vi "FeedbackDecode.vi"() -> ()   [LabVIEW 2020] (continued)
            n2364 = call "FeedbackDecode_MLComCtrl.vi"("DecodeClustIn"=w2568, "Mode"=T19."SendEvent") -> ()  [unwired: 6 in, 4 out]
          }
          event Value Change {
            n2365 = event-data() -> ()  [unwired: 1 in, 6 out]
            n2366 = local read "EncodeClust"() -> (w2595:T9)
            n2367 = call "FeedbackDecode_BuildStimCmd.vi"("EncodeClustIn"=w2595) -> ("EncodeClustOut"=w2594:T9, "StimCmd"=w2579:string)  [unwired: 1 in]
            n2368 = local read "LoopCnt"() -> (w2589:u64)
            n2369 = local write "EncodeClust"(w2594) -> ()
            n2370 = local read "NIPTime"() -> (w2585:dbl)
            n2371 = Format Into String(w2589) -> (resulting string=w2580:string)  [unwired: 3 in, 1 out]
            n2372 = call-poly "FeedbackDecode_VariablesToString.vi"("Format"="%0.0f", "ValueIn"=w2585, "FieldName"="NIPTime" ("Key Word")) -> ("StringOut"=w2582:string)  [unwired: 4 in]
            n2373 = local read "EventParamsFID"() -> (w2592:refnum<file>)
            n2374 = Concatenate Strings("ChangeJitter:SS.EventID=" ("string"), w2580) -> (w2588:string)
            n2375 = local write "StimCmd"(w2579) -> ()
            n2376 = Concatenate Strings(w2588, ";", w2579, w2582) -> (w2587:string)
            n2377 = local read "DecodeClust"() -> (w2593:T5)
            n2378 = call "FeedbackDecode_WriteTextEOL.vi"("text"=w2587, "refnum in"=w2592) -> ()  [unwired: 8 in, 2 out]
            n2379 = Bundle By Name(cluster=w2593, "EventStr"=w2587) -> (w2586:T5)
            n2380 = call "FeedbackDecode_MLComCtrl.vi"("DecodeClustIn"=w2586, "Mode"=T19."SendEvent") -> ()  [unwired: 6 in, 4 out]
          }
          event Value Change {
            n2381 = event-data() -> ()  [unwired: 1 in, 6 out]
            n2382 = local read "EncodeClust"() -> (w2613:T9)
            n2383 = call "FeedbackDecode_BuildStimCmd.vi"("EncodeClustIn"=w2613) -> ("EncodeClustOut"=w2612:T9, "StimCmd"=w2597:string)  [unwired: 1 in]
            n2384 = local read "LoopCnt"() -> (w2607:u64)
            n2385 = local write "EncodeClust"(w2612) -> ()
            n2386 = local read "NIPTime"() -> (w2603:dbl)
            n2387 = Format Into String(w2607) -> (resulting string=w2598:string)  [unwired: 3 in, 1 out]
            n2388 = call-poly "FeedbackDecode_VariablesToString.vi"("Format"="%0.0f", "ValueIn"=w2603, "FieldName"="NIPTime" ("Key Word")) -> ("StringOut"=w2600:string)  [unwired: 4 in]
            n2389 = Concatenate Strings("ChangeBFreq:SS.EventID=" ("string"), w2598) -> (w2606:string)
            n2390 = local read "EventParamsFID"() -> (w2610:refnum<file>)
            n2391 = local write "StimCmd"(w2597) -> ()
            n2392 = Concatenate Strings(w2606, ";", w2597, w2600) -> (w2605:string)
            n2393 = local read "DecodeClust"() -> (w2611:T5)
            n2394 = call "FeedbackDecode_WriteTextEOL.vi"("text"=w2605, "refnum in"=w2610) -> ()  [unwired: 8 in, 2 out]
            n2395 = Bundle By Name(cluster=w2611, "EventStr"=w2605) -> (w2604:T5)
            n2396 = call "FeedbackDecode_MLComCtrl.vi"("DecodeClustIn"=w2604, "Mode"=T19."SendEvent") -> ()  [unwired: 6 in, 4 out]
          }
          event Value Change {
            n2397 = event-data() -> ()  [unwired: 1 in, 6 out]
            n2398 = local read "EncodeClust"() -> (w2631:T9)
            n2399 = call "FeedbackDecode_BuildStimCmd.vi"("EncodeClustIn"=w2631) -> ("EncodeClustOut"=w2630:T9, "StimCmd"=w2615:string)  [unwired: 1 in]
            n2400 = local read "LoopCnt"() -> (w2625:u64)
            n2401 = local write "EncodeClust"(w2630) -> ()
            n2402 = local read "NIPTime"() -> (w2621:dbl)
            n2403 = Format Into String(w2625) -> (resulting string=w2616:string)  [unwired: 3 in, 1 out]
            n2404 = call-poly "FeedbackDecode_VariablesToString.vi"("Format"="%0.0f", "ValueIn"=w2621, "FieldName"="NIPTime" ("Key Word")) -> ("StringOut"=w2618:string)  [unwired: 4 in]
            n2405 = local read "EventParamsFID"() -> (w2628:refnum<file>)
            n2406 = Concatenate Strings("ChangeBAmp:SS.EventID=" ("string"), w2616) -> (w2624:string)
            n2407 = local write "StimCmd"(w2615) -> ()
            n2408 = local read "DecodeClust"() -> (w2629:T5)
            n2409 = Concatenate Strings(w2624, ";", w2615, w2618) -> (w2623:string)
            n2410 = call "FeedbackDecode_WriteTextEOL.vi"("text"=w2623, "refnum in"=w2628) -> ()  [unwired: 8 in, 2 out]
            n2411 = Bundle By Name(cluster=w2629, "EventStr"=w2623) -> (w2622:T5)
            n2412 = call "FeedbackDecode_MLComCtrl.vi"("DecodeClustIn"=w2622, "Mode"=T19."SendEvent") -> ()  [unwired: 6 in, 4 out]
          }
          event "TASKA Shared Control": Value Change {
            n2413 = event-data() -> ("NewVal"=w2635:bool)  [unwired: 1 in, 5 out]
            n2414 = case shown="True" w2635 {
              tunnel: [0.0 1.0] -> w2634
              frame False {
              }
              frame True {
              }
            }
            n2415 = local read "LoopCnt"() -> (w2644:u64)
            n2416 = call-poly "FeedbackDecode_VariablesToString.vi"("Format"="%d", "ValueIn"=w2634, "FieldName"="TASKASensors.SharedControl.Ready") -> ("StringOut"=w2651:string)  [unwired: 4 in]
            n2417 = local read "NIPTime"() -> (w2640:dbl)
            n2418 = Format Into String(w2644) -> (resulting string=w2636:string)  [unwired: 3 in, 1 out]
            n2419 = local read "EventParamsFID"() -> (w2648:refnum<file>)
            n2420 = local read "DecodeClust"() -> (w2649:T5)
            n2421 = Concatenate Strings("SharedControl:SS.EventID=" ("string"), w2636) -> (w2643:string)
            n2422 = call-poly "FeedbackDecode_VariablesToString.vi"("Format"="%0.0f", "ValueIn"=w2640, "FieldName"="NIPTime" ("Key Word")) -> ("StringOut"=w2637:string)  [unwired: 4 in]
            n2423 = Concatenate Strings(w2643, ";", w2651, w2637) -> (w2642:string)
            n2424 = call "FeedbackDecode_WriteTextEOL.vi"("text"=w2642, "refnum in"=w2648) -> ()  [unwired: 8 in, 2 out]
            n2425 = Bundle By Name(cluster=w2649, "EventStr"=w2642) -> (w2641:T5)
            n2426 = call "FeedbackDecode_MLComCtrl.vi"("DecodeClustIn"=w2641, "Mode"=T19."SendEvent") -> ()  [unwired: 6 in, 4 out]
          }
          event "TASKA Timer": Value Change {
            n2427 = event-data() -> ("NewVal"=w2655:bool)  [unwired: 1 in, 5 out]
            n2428 = case shown="True" w2655 {
              frame True {
                n2429 = local read "LoopCnt"() -> (w2660:u64)
                n2430 = local read "NIPTime"() -> (w2663:dbl)
                n2431 = Format Into String(w2660) -> (resulting string=w2667:string)  [unwired: 3 in, 1 out]
                n2432 = local read "EventParamsFID"() -> (w2657:refnum<file>)
                n2433 = Concatenate Strings("SharedControlStartTime:SS.EventID=" ("string"), w2667) -> (w2661:string)
                n2434 = call-poly "FeedbackDecode_VariablesToString.vi"("Format"="%0.0f", "ValueIn"=w2663, "FieldName"="NIPTime" ("Key Word")) -> ("StringOut"=w2666:string)  [unwired: 4 in]
                n2435 = Concatenate Strings(w2661, ";", w2666) -> (w2662:string)
                n2436 = call "FeedbackDecode_WriteTextEOL.vi"("text"=w2662, "refnum in"=w2657) -> ()  [unwired: 8 in, 2 out]
              }
              frame False {
                n2437 = property on="TASKA Timer" class="Bool (strict)"("DisabledEnum"=T17."Disabled and Grayed Out" ("Disabled")) -> ()  [unwired: 2 in, 2 out]
                n2438 = local read "LoopCnt"() -> (w2672:u64)
                n2439 = local read "NIPTime"() -> (w2675:dbl)
                n2440 = Format Into String(w2672) -> (resulting string=w2679:string)  [unwired: 3 in, 1 out]
                n2441 = local read "EventParamsFID"() -> (w2669:refnum<file>)
                n2442 = Concatenate Strings("SharedControlStopTime:SS.EventID=" ("string"), w2679) -> (w2673:string)
                n2443 = call-poly "FeedbackDecode_VariablesToString.vi"("Format"="%0.0f", "ValueIn"=w2675, "FieldName"="NIPTime" ("Key Word")) -> ("StringOut"=w2678:string)  [unwired: 4 in]
                n2444 = Concatenate Strings(w2673, ";", w2678) -> (w2674:string)
                n2445 = call "FeedbackDecode_WriteTextEOL.vi"("text"=w2674, "refnum in"=w2669) -> ()  [unwired: 8 in, 2 out]
              }
            }
          }
          event "TASKA Reset Break": Value Change {
            n2446 = event-data() -> ()  [unwired: 1 in, 6 out]
            n2447 = call-poly "FeedbackDecode_VariablesToString.vi"("Format"="%0.0f", "ValueIn"=0.0, "FieldName"="SharedControlTrialSuccess" ("Key Word")) -> ("StringOut"=w2681:string)  [unwired: 4 in]
            n2448 = property on="TASKA Timer" class="Bool (strict)"("DisabledEnum"=T17."Enabled" ("Disabled")) -> ()  [unwired: 2 in, 2 out]
            n2449 = local read "LoopCnt"() -> (w2688:u64)
            n2450 = local read "NIPTime"() -> (w2691:dbl)
            n2451 = Format Into String(w2688) -> (resulting string=w2695:string)  [unwired: 3 in, 1 out]
            n2452 = local read "EventParamsFID"() -> (w2685:refnum<file>)
            n2453 = Concatenate Strings("SharedControlTrialResult:SS.EventID=" ("string"), w2695) -> (w2689:string)
            n2454 = call-poly "FeedbackDecode_VariablesToString.vi"("Format"="%0.0f", "ValueIn"=w2691, "FieldName"="NIPTime" ("Key Word")) -> ("StringOut"=w2694:string)  [unwired: 4 in]
            n2455 = Concatenate Strings(w2689, ";", w2681, w2694) -> (w2690:string)
            n2456 = call "FeedbackDecode_WriteTextEOL.vi"("text"=w2690, "refnum in"=w2685) -> ()  [unwired: 8 in, 2 out]
          }
          event "TASKA Reset Success": Value Change {
            n2457 = event-data() -> ()  [unwired: 1 in, 6 out]
            n2458 = call-poly "FeedbackDecode_VariablesToString.vi"("Format"="%0.0f", "ValueIn"=1.0, "FieldName"="SharedControlTrialSuccess" ("Key Word")) -> ("StringOut"=w2698:string)  [unwired: 4 in]
            n2459 = property on="TASKA Timer" class="Bool (strict)"("DisabledEnum"=T17."Enabled" ("Disabled")) -> ()  [unwired: 2 in, 2 out]
            n2460 = local read "LoopCnt"() -> (w2705:u64)
            n2461 = local read "NIPTime"() -> (w2708:dbl)
            n2462 = Format Into String(w2705) -> (resulting string=w2712:string)  [unwired: 3 in, 1 out]
            n2463 = local read "EventParamsFID"() -> (w2702:refnum<file>)
            n2464 = Concatenate Strings("SharedControlTrialResult:SS.EventID=" ("string"), w2712) -> (w2706:string)
            n2465 = call-poly "FeedbackDecode_VariablesToString.vi"("Format"="%0.0f", "ValueIn"=w2708, "FieldName"="NIPTime" ("Key Word")) -> ("StringOut"=w2711:string)  [unwired: 4 in]
            n2466 = Concatenate Strings(w2706, ";", w2698, w2711) -> (w2707:string)
            n2467 = call "FeedbackDecode_WriteTextEOL.vi"("text"=w2707, "refnum in"=w2702) -> ()  [unwired: 8 in, 2 out]
          }
          event "TASKASharedControlBeta": Value Change {
            n2468 = event-data() -> ("NewVal"=w2714:dbl)  [unwired: 1 in, 5 out]
            n2469 = local read "LoopCnt"() -> (w2724:u64)
            n2470 = call-poly "FeedbackDecode_VariablesToString.vi"("Format"="%0.5f", "ValueIn"=w2714, "FieldName"="TASKASensors.SharedControl.Beta") -> ("StringOut"=w2731:string)  [unwired: 4 in]
            n2471 = local read "NIPTime"() -> (w2720:dbl)
            n2472 = Format Into String(w2724) -> (resulting string=w2716:string)  [unwired: 3 in, 1 out]
            n2473 = local read "EventParamsFID"() -> (w2728:refnum<file>)
            n2474 = local read "DecodeClust"() -> (w2729:T5)
            n2475 = Concatenate Strings("SharedControl:SS.EventID=" ("string"), w2716) -> (w2723:string)
            n2476 = call-poly "FeedbackDecode_VariablesToString.vi"("Format"="%0.0f", "ValueIn"=w2720, "FieldName"="NIPTime" ("Key Word")) -> ("StringOut"=w2717:string)  [unwired: 4 in]
            n2477 = Concatenate Strings(w2723, ";", w2731, w2717) -> (w2722:string)
            n2478 = call "FeedbackDecode_WriteTextEOL.vi"("text"=w2722, "refnum in"=w2728) -> ()  [unwired: 8 in, 2 out]
            n2479 = Bundle By Name(cluster=w2729, "EventStr"=w2722) -> (w2721:T5)
            n2480 = call "FeedbackDecode_MLComCtrl.vi"("DecodeClustIn"=w2721, "Mode"=T19."SendEvent") -> ()  [unwired: 6 in, 4 out]
          }
          event "TASKASharedControlIncrememnt": Value Change {
            n2481 = event-data() -> ("NewVal"=w2733:dbl)  [unwired: 1 in, 5 out]
            n2482 = local read "LoopCnt"() -> (w2743:u64)
            n2483 = call-poly "FeedbackDecode_VariablesToString.vi"("Format"="%0.5f", "ValueIn"=w2733, "FieldName"="TASKASensors.SharedControl.Increment") -> ("StringOut"=w2750:string)  [unwired: 4 in]
            n2484 = local read "NIPTime"() -> (w2739:dbl)
            n2485 = Format Into String(w2743) -> (resulting string=w2735:string)  [unwired: 3 in, 1 out]
            n2486 = local read "EventParamsFID"() -> (w2747:refnum<file>)
            n2487 = local read "DecodeClust"() -> (w2748:T5)
            n2488 = Concatenate Strings("SharedControl:SS.EventID=" ("string"), w2735) -> (w2742:string)
            n2489 = call-poly "FeedbackDecode_VariablesToString.vi"("Format"="%0.0f", "ValueIn"=w2739, "FieldName"="NIPTime" ("Key Word")) -> ("StringOut"=w2736:string)  [unwired: 4 in]
            n2490 = Concatenate Strings(w2742, ";", w2750, w2736) -> (w2741:string)
            n2491 = call "FeedbackDecode_WriteTextEOL.vi"("text"=w2741, "refnum in"=w2747) -> ()  [unwired: 8 in, 2 out]
            n2492 = Bundle By Name(cluster=w2748, "EventStr"=w2741) -> (w2740:T5)
            n2493 = call "FeedbackDecode_MLComCtrl.vi"("DecodeClustIn"=w2740, "Mode"=T19."SendEvent") -> ()  [unwired: 6 in, 4 out]
          }
          event "IndexSet", "MiddleSet", "RingSet", "PinkySet", "ThumbSet", "ThumbIntSet": Value Change {
            n2494 = event-data() -> ()  [unwired: 1 in, 6 out]
            n2495 = local read "ThumbIntSet"() -> (w2752:dbl)
            n2496 = local read "ThumbSet"() -> (w2753:dbl)
            n2497 = local read "MiddleSet"() -> (w2758:dbl)
            n2498 = local read "RingSet"() -> (w2757:dbl)
            n2499 = local read "PinkySet"() -> (w2754:dbl)
            n2500 = local read "IndexSet"() -> (w2759:dbl)
            n2501 = Build Array(w2759, w2758, w2757, w2754, w2753, w2752) -> (w2756:dbl[])
            n2502 = local read "LoopCnt"() -> (w2768:u64)
            n2503 = call-poly "FeedbackDecode_VariablesToString.vi"("Format"="%0.5f", "ValueIn"=w2756, "FieldName"="TASKA.RestPositions") -> ("StringOut"=w2775:string)  [unwired: 4 in]
            n2504 = local read "NIPTime"() -> (w2764:dbl)
            n2505 = Format Into String(w2768) -> (resulting string=w2761:string)  [unwired: 3 in, 1 out]
            n2506 = local read "EventParamsFID"() -> (w2772:refnum<file>)
            n2507 = local read "DecodeClust"() -> (w2773:T5)
            n2508 = Concatenate Strings("SharedControl:SS.EventID=" ("string"), w2761) -> (w2767:string)
            n2509 = call-poly "FeedbackDecode_VariablesToString.vi"("Format"="%0.0f", "ValueIn"=w2764, "FieldName"="NIPTime" ("Key Word")) -> ("StringOut"=w2755:string)  [unwired: 4 in]
            n2510 = Concatenate Strings(w2767, ";", w2775, w2755) -> (w2766:string)
            n2511 = call "FeedbackDecode_WriteTextEOL.vi"("text"=w2766, "refnum in"=w2772) -> ()  [unwired: 8 in, 2 out]
            n2512 = Bundle By Name(cluster=w2773, "EventStr"=w2766) -> (w2765:T5)
            n2513 = call "FeedbackDecode_MLComCtrl.vi"("DecodeClustIn"=w2765, "Mode"=T19."SendEvent") -> ()  [unwired: 6 in, 4 out]
          }
          event "ThumbShare", "IndexShare", "MiddleShare", "RingShare": Value Change {
            n2514 = event-data() -> ()  [unwired: 1 in, 6 out]
            n2515 = local read "ThumbShare"() -> (w2780:bool)
            n2516 = local read "MiddleShare"() -> (w2784:bool)
            n2517 = local read "RingShare"() -> (w2783:bool)
            n2518 = local read "IndexShare"() -> (w2785:bool)
            n2519 = Build Array(w2785, w2784, w2783, FALSE ("element"), w2780, FALSE ("element")) -> (w2778:bool[])
            n2520 = for {
              tunnel: w2778 -> [w2804] mode=indexing
              tunnel: [w2803] -> w2777 mode=indexing
              n2521 = case shown="False" w2804 {
                tunnel: [0.0 ("ValueIn") 1.0 ("ValueIn")] -> w2803
                frame False {
                }
                frame True {
                }
              }
            }
            n2522 = local read "LoopCnt"() -> (w2794:u64)
            n2523 = local read "NIPTime"() -> (w2790:dbl)
            n2524 = call-poly "FeedbackDecode_VariablesToString.vi"("Format"="%1.0f", "ValueIn"=w2777, "FieldName"="TASKASensors.SharedEnabled") -> ("StringOut"=w2801:string)  [unwired: 4 in]
            n2525 = Format Into String(w2794) -> (resulting string=w2787:string)  [unwired: 3 in, 1 out]
            n2526 = local read "EventParamsFID"() -> (w2798:refnum<file>)
            n2527 = local read "DecodeClust"() -> (w2799:T5)
            n2528 = Concatenate Strings("SharedControl:SS.EventID=" ("string"), w2787) -> (w2793:string)
            n2529 = call-poly "FeedbackDecode_VariablesToString.vi"("Format"="%0.0f", "ValueIn"=w2790, "FieldName"="NIPTime" ("Key Word")) -> ("StringOut"=w2782:string)  [unwired: 4 in]
            n2530 = Concatenate Strings(w2793, ";", w2801, w2782) -> (w2792:string)
            n2531 = call "FeedbackDecode_WriteTextEOL.vi"("text"=w2792, "refnum in"=w2798) -> ()  [unwired: 8 in, 2 out]
            n2532 = Bundle By Name(cluster=w2799, "EventStr"=w2792) -> (w2791:T5)
            n2533 = call "FeedbackDecode_MLComCtrl.vi"("DecodeClustIn"=w2791, "Mode"=T19."SendEvent") -> ()  [unwired: 6 in, 4 out]
          }
          event "Computer Goal": Value Change {
            n2534 = event-data() -> ("NewVal"=w2807:string)  [unwired: 1 in, 5 out]
            n2535 = local read "LoopCnt"() -> (w2817:u64)
            n2536 = call-poly "FeedbackDecode_VariablesToString.vi"("Format"="%0.5f", "ValueIn"=w2807, "FieldName"="TASKASensors.SharedControl.ComputerGoal") -> ("StringOut"=w2824:string)  [unwired: 4 in]
            n2537 = local read "NIPTime"() -> (w2813:dbl)
            n2538 = Format Into String(w2817) -> (resulting string=w2809:string)  [unwired: 3 in, 1 out]
            n2539 = local read "EventParamsFID"() -> (w2821:refnum<file>)
            n2540 = local read "DecodeClust"() -> (w2822:T5)
            n2541 = Concatenate Strings("SharedControl:SS.EventID=" ("string"), w2809) -> (w2816:string)
            n2542 = call-poly "FeedbackDecode_VariablesToString.vi"("Format"="%0.0f", "ValueIn"=w2813, "FieldName"="NIPTime" ("Key Word")) -> ("StringOut"=w2810:string)  [unwired: 4 in]
            n2543 = Concatenate Strings(w2816, ";", w2824, w2810) -> (w2815:string)
            n2544 = call "FeedbackDecode_WriteTextEOL.vi"("text"=w2815, "refnum in"=w2821) -> ()  [unwired: 8 in, 2 out]
            n2545 = Bundle By Name(cluster=w2822, "EventStr"=w2815) -> (w2814:T5)
            n2546 = call "FeedbackDecode_MLComCtrl.vi"("DecodeClustIn"=w2814, "Mode"=T19."SendEvent") -> ()  [unwired: 6 in, 4 out]
          }
          event "Beta Mode": Value Change {
            n2547 = event-data() -> ("NewVal"=w2826:string)  [unwired: 1 in, 5 out]
            n2548 = local read "LoopCnt"() -> (w2836:u64)
            n2549 = call-poly "FeedbackDecode_VariablesToString.vi"("Format"="%0.5f", "ValueIn"=w2826, "FieldName"="TASKASensors.SharedControl.BetaMode") -> ("StringOut"=w2843:string)  [unwired: 4 in]
            n2550 = local read "NIPTime"() -> (w2832:dbl)
            n2551 = Format Into String(w2836) -> (resulting string=w2828:string)  [unwired: 3 in, 1 out]
            n2552 = local read "EventParamsFID"() -> (w2840:refnum<file>)
            n2553 = local read "DecodeClust"() -> (w2841:T5)
            n2554 = Concatenate Strings("SharedControl:SS.EventID=" ("string"), w2828) -> (w2835:string)
            n2555 = call-poly "FeedbackDecode_VariablesToString.vi"("Format"="%0.0f", "ValueIn"=w2832, "FieldName"="NIPTime" ("Key Word")) -> ("StringOut"=w2829:string)  [unwired: 4 in]
            n2556 = Concatenate Strings(w2835, ";", w2843, w2829) -> (w2834:string)
            n2557 = call "FeedbackDecode_WriteTextEOL.vi"("text"=w2834, "refnum in"=w2840) -> ()  [unwired: 8 in, 2 out]
            n2558 = Bundle By Name(cluster=w2841, "EventStr"=w2834) -> (w2833:T5)
            n2559 = call "FeedbackDecode_MLComCtrl.vi"("DecodeClustIn"=w2833, "Mode"=T19."SendEvent") -> ()  [unwired: 6 in, 4 out]
          }
          event Mouse Wheel; Mouse Down; Mouse Move {
            n2560 = event-data() -> ("CtlRef"=w2845:refnum<vi>)  [unwired: 1 in, 4 out]
            n2561 = property class="Arr (strict)"(reference=w2845) -> ("Index Values"=w2846:u32[])  [unwired: 1 in, 2 out]
            n2562 = Index Array(array=w2846) -> (element=w2847:u32)  [unwired: 1 in]
            n2563 = Build Array(w2847) -> (w2848:u32[])
            n2564 = property on="Sel" class="Arr (strict)"("Index Values"=w2848) -> ()  [unwired: 2 in, 2 out]
          }
          event "RespStr": Value Change {
            n2565 = event-data() -> ("NewVal"=w2850:string)  [unwired: 1 in, 5 out]
            n2566 = Empty String/Path?(string/path=w2850) -> (empty?=w2851:bool)
            n2567 = case shown="False" w2851 {
              tunnel: w2850 -> [w2855 _]
              frame False {
                n2568 = xnode "Match Regular Expression"("input string"=w2855, "regular expression"="Sensor='") -> ("after match"=w2858:string)  [unwired: 4 in, 4 out]
                n2569 = local read "EncodeClust"() -> (w2860:T9)
                n2570 = xnode "Match Regular Expression"("input string"=w2858, "regular expression"="';") -> ("before match"=w2854:string)  [unwired: 4 in, 4 out]
                n2571 = call "FeedbackDecode_UpdateRegion.vi"("EncodeClustIn"=w2860, "RegionStr"=w2854) -> ("EncodeClustOut"=w2859:T9)  [unwired: 1 in]
                n2572 = local write "EncodeClust"(w2859) -> ()
                n2573 = local read "LoopCnt"() -> (w2870:u64)
                n2574 = local read "NIPTime"() -> (w2866:dbl)
                n2575 = local read "StimCmd"() -> (w2853:string)
                n2576 = Format Into String(w2870) -> (resulting string=w2861:string)  [unwired: 3 in, 1 out]
                n2577 = call-poly "FeedbackDecode_VariablesToString.vi"("Format"="%0.0f", "ValueIn"=w2866, "FieldName"="NIPTime" ("Key Word")) -> ("StringOut"=w2863:string)  [unwired: 4 in]
                n2578 = Concatenate Strings("Response:SS.EventID=" ("string"), w2861) -> (w2869:string)
                n2579 = local read "EventParamsFID"() -> (w2873:refnum<file>)
                n2580 = Concatenate Strings(w2869, ";", w2855, w2853, w2863) -> (w2868:string)
                n2581 = local read "DecodeClust"() -> (w2874:T5)
                n2582 = call "FeedbackDecode_WriteTextEOL.vi"("text"=w2868, "refnum in"=w2873) -> ()  [unwired: 8 in, 2 out]
                n2583 = Bundle By Name(cluster=w2874, "EventStr"=w2868) -> (w2867:T5)
                n2584 = call "FeedbackDecode_MLComCtrl.vi"("DecodeClustIn"=w2867, "Mode"=T19."SendEvent") -> ()  [unwired: 6 in, 4 out]
              }
              frame True {
              }
            }
          }
          event Value Change {
            n2585 = event-data() -> ("NewVal"=w3103:bool)  [unwired: 1 in, 5 out]
            n2586 = case shown="True" w3103 {
              frame False {
              }
              frame True {
                n2587 = local read "EncodeClust"() -> (w3107:T9)
                n2588 = Bundle By Name(cluster=w3107, "RespClust.OpenResp"=FALSE ("OpenResp")) -> (w3109:T9)
                n2589 = local read "RespRefArray"() -> (w3108:refnum<vi>[])
                n2590 = local write "EncodeClust"(w3109) -> ()
                n2591 = Unbundle By Name(w3107) -> ("RespClust.RespType"=w3106:enum16{"Sensor Map", "Full Map"})
                n2592 = Index Array(array=w3108, index=w3106) -> (element=w3105:refnum<vi>)
                n2593 = invoke class="VI" method="FP.Open"(reference=w3105, "Activate"=TRUE ("Activate?"), "State"=T21."Standard") -> (reference out=w3114:refnum<vi>)  [unwired: 2 in, 4 out]
                n2594 = property class="VI"(reference=w3114, "Front Panel.IsFrontmost"=TRUE ("Front Panel Window:Is Frontmost")) -> ()  [unwired: 1 in, 2 out]
                n2595 = local read "LoopCnt"() -> (w3124:u64)
                n2596 = local read "NIPTime"() -> (w3120:dbl)
                n2597 = Format Into String(w3124) -> (resulting string=w3115:string)  [unwired: 3 in, 1 out]
                n2598 = call-poly "FeedbackDecode_VariablesToString.vi"("Format"="%0.0f", "ValueIn"=w3120, "FieldName"="NIPTime" ("Key Word")) -> ("StringOut"=w3117:string)  [unwired: 4 in]
                n2599 = Concatenate Strings("OpenResp:SS.EventID=" ("string"), w3115) -> (w3123:string)
                n2600 = local read "EventParamsFID"() -> (w3127:refnum<file>)
                n2601 = Concatenate Strings(w3123, ";", w3117) -> (w3122:string)
                n2602 = local read "DecodeClust"() -> (w3128:T5)
                n2603 = call "FeedbackDecode_WriteTextEOL.vi"("text"=w3122, "refnum in"=w3127) -> ()  [unwired: 8 in, 2 out]
                n2604 = Bundle By Name(cluster=w3128, "EventStr"=w3122) -> (w3121:T5)
                n2605 = call "FeedbackDecode_MLComCtrl.vi"("DecodeClustIn"=w3121, "Mode"=T19."SendEvent") -> ()  [unwired: 6 in, 4 out]
              }
            }
          }
          event Value Change {
            n2606 = event-data() -> ("NewVal"=w3153:T52)  [unwired: 1 in, 5 out]
            n2607 = Cluster To Array(cluster=w3153) -> (array=w3152:bool[])
            n2608 = Search 1D Array(1D array=w3152, element=TRUE) -> (index of element=w3129:i32)  [unwired: 1 in]
            n2609 = local read "EncodeClust"() -> (w3130:T9)
            n2610 = call "FeedbackDecode_SortParamsTable.vi"("StimClustIn"=w3130, "Column"=w3129) -> ("StimClustOut"=w3150:T9)  [unwired: 1 in]
            n2611 = call "FeedbackDecode_Params2Preset.vi"("StimClustIn"=w3150) -> ("StimClustOut"=w3149:T9)  [unwired: 2 in]
            n2612 = local read "LoopCnt"() -> (w3141:u64)
            n2613 = call "FeedbackDecode_UpdateParamsTable.vi"("StimClustIn"=w3149) -> ("StimClustOut"=w3148:T9)  [unwired: 2 in]
            n2614 = call "FeedbackDecode_Params2UEA.vi"("StimClustIn"=w3148) -> ("StimClustOut"=w3147:T9)  [unwired: 2 in]
            n2615 = Format Into String(w3141) -> (resulting string=w3133:string)  [unwired: 3 in, 1 out]
            n2616 = local read "NIPTime"() -> (w3137:dbl)
            n2617 = call "FeedbackDecode_BuildStimCmd.vi"("EncodeClustIn"=w3147) -> ("EncodeClustOut"=w3132:T9, "StimCmd"=w3131:string)  [unwired: 1 in]
            n2618 = local read "EventParamsFID"() -> (w3145:refnum<file>)
            n2619 = Concatenate Strings("SortStim:SS.EventID=" ("string"), w3133) -> (w3140:string)
            n2620 = call-poly "FeedbackDecode_VariablesToString.vi"("Format"="%0.0f", "ValueIn"=w3137, "FieldName"="NIPTime" ("Key Word")) -> ("StringOut"=w3134:string)  [unwired: 4 in]
            n2621 = local read "DecodeClust"() -> (w3146:T5)
            n2622 = Concatenate Strings(w3140, ";", w3131, w3134) -> (w3139:string)
            n2623 = call "FeedbackDecode_WriteTextEOL.vi"("text"=w3139, "refnum in"=w3145) -> ()  [unwired: 8 in, 2 out]
            n2624 = Bundle By Name(cluster=w3146, "EventStr"=w3139) -> (w3138:T5)
            n2625 = local write "StimCmd"(w3131) -> ()
            n2626 = local write "EncodeClust"(w3132) -> ()
            n2627 = call "FeedbackDecode_MLComCtrl.vi"("DecodeClustIn"=w3138, "Mode"=T19."SendEvent") -> ()  [unwired: 6 in, 4 out]
          }
          event Value Change {
            n2628 = event-data() -> ()  [unwired: 1 in, 6 out]
            n2629 = local read "EncodeClust"() -> (w3156:T9)
            n2630 = Unbundle By Name(w3156) -> ("Sel"=w3157:bool[])
            n2631 = local read "SelTog"() -> (w3160:bool)
            n2632 = case shown="False" w3160 {
              selector: w3160 -> [w3182 w3188]
              tunnel: w3157 -> [w3186 w3192]
              tunnel: [w3183 w3189] -> w3158
              frame True {
                n2633 = Not(x=w3182) -> (.not. x?=w3181:bool)
                n2634 = Array Size(array=w3186) -> (size(s)=w3185:i32)
                n2635 = local write "SelTog"(w3181) -> ()
                n2636 = Initialize Array(FALSE, w3185) -> (w3183:bool[])
              }
              frame False {
                n2637 = Not(x=w3188) -> (.not. x?=w3187:bool)
                n2638 = Array Size(array=w3192) -> (size(s)=w3191:i32)
                n2639 = local write "SelTog"(w3187) -> ()
                n2640 = Initialize Array(TRUE, w3191) -> (w3189:bool[])
              }
            }
            n2641 = Bundle By Name(cluster=w3156, "Sel"=w3158, "SelSort.Sel"=FALSE) -> (w3155:T9)
            n2642 = call "FeedbackDecode_Params2Preset.vi"("StimClustIn"=w3155) -> ("StimClustOut"=w3179:T9)  [unwired: 2 in]
            n2643 = local read "LoopCnt"() -> (w3171:u64)
            n2644 = call "FeedbackDecode_UpdateParamsTable.vi"("StimClustIn"=w3179) -> ("StimClustOut"=w3178:T9)  [unwired: 2 in]
            n2645 = call "FeedbackDecode_Params2UEA.vi"("StimClustIn"=w3178) -> ("StimClustOut"=w3177:T9)  [unwired: 2 in]
            n2646 = Format Into String(w3171) -> (resulting string=w3163:string)  [unwired: 3 in, 1 out]
            n2647 = local read "NIPTime"() -> (w3167:dbl)
            n2648 = call "FeedbackDecode_BuildStimCmd.vi"("EncodeClustIn"=w3177) -> ("EncodeClustOut"=w3162:T9, "StimCmd"=w3161:string)  [unwired: 1 in]
            n2649 = local read "EventParamsFID"() -> (w3175:refnum<file>)
            n2650 = Concatenate Strings("SortStim:SS.EventID=" ("string"), w3163) -> (w3170:string)
            n2651 = call-poly "FeedbackDecode_VariablesToString.vi"("Format"="%0.0f", "ValueIn"=w3167, "FieldName"="NIPTime" ("Key Word")) -> ("StringOut"=w3164:string)  [unwired: 4 in]
            n2652 = local read "DecodeClust"() -> (w3176:T5)
            n2653 = Concatenate Strings(w3170, ";", w3161, w3164) -> (w3169:string)
            n2654 = call "FeedbackDecode_WriteTextEOL.vi"("text"=w3169, "refnum in"=w3175) -> ()  [unwired: 8 in, 2 out]
            n2655 = Bundle By Name(cluster=w3176, "EventStr"=w3169) -> (w3168:T5)
            n2656 = local write "StimCmd"(w3161) -> ()
            n2657 = local write "EncodeClust"(w3162) -> ()
            n2658 = call "FeedbackDecode_MLComCtrl.vi"("DecodeClustIn"=w3168, "Mode"=T19."SendEvent") -> ()  [unwired: 6 in, 4 out]
          }
          event Key Down {
            n2659 = event-data() -> ("Char"=w3194:i16, "VKey"=w3195:T53)  [unwired: 1 in, 8 out]
            n2660 = local read "LVTab"() -> (w3193:T4)
            n2661 = case shown="\"Encode\"" w3193 {
              tunnel: w3195 -> [_ w3198]
              tunnel: w3194 -> [_ w3197]
              frame "Decode", Default {
              }
              frame "Encode" {
                n2662 = case shown="\"Up\"" w3198 {
                  tunnel: w3197 -> [w3199 _ _ _ _ _]
                  frame "ASCII" {
                    n2663 = case shown="115" w3199 {
                      frame -1, Default {
                      }
                      frame 115 {
                        # "s=stim"
                        n2664 = disable-structure shown="Disabled" {
                          frame Disabled {
                            n2665 = local read "StimTog"() -> (w3200:bool)
                            n2666 = case shown="True" w3200 {
                              selector: w3200 -> [w3202 w3204]
                              frame True {
                                n2667 = Not(x=w3202) -> (.not. x?=w3201:bool)
                                n2668 = local write "StimTog"(w3201) -> ()
                                n2669 = property on="Stim" class="Bool (strict)"("Val(Sgnl)"=w3201) -> ()  [unwired: 2 in, 2 out]
                              }
                              frame False {
                                n2670 = Not(x=w3204) -> (.not. x?=w3203:bool)
                                n2671 = local write "StimTog"(w3203) -> ()
                                n2672 = property on="Stim" class="Bool (strict)"("Val(Sgnl)"=w3203) -> ()  [unwired: 2 in, 2 out]
                              }
                            }
                          }
                          frame Enabled {
                          }
                        }
                      }
                    }
                  }
                  frame Default {
                  }
                  frame "Up" {
                    n2673 = property on="Add" class="Bool (strict)"("Val(Sgnl)"=TRUE ("Value (Signaling)")) -> ()  [unwired: 2 in, 2 out]
                  }
                  frame "Down" {
                    n2674 = property on="Sub" class="Bool (strict)"("Val(Sgnl)"=TRUE ("Value (Signaling)")) -> ()  [unwired: 2 in, 2 out]
                  }
                  frame "Left" {
                    w3212 = 100 ("length")
                    n2675 = local read "EncodeClust"() -> (w3225:T9)
                    n2676 = Unbundle By Name(w3225) -> ("UEAArray"=w3220:T25)
                    n2677 = Index Array(array=w3220) -> (element #1=w3221:T54, element #2=w3222:T54)  [unwired: 2 in]
                    n2678 = Cluster To Array(cluster=w3221) -> (array=w3223:bool[])
                    n2679 = Cluster To Array(cluster=w3222) -> (array=w3224:bool[])
                    n2680 = Build Array (concatenate)(w3223, w3224) -> (w3219:bool[])
                    n2681 = Search 1D Array(1D array=w3219, element=TRUE) -> (index of element=w3216:i32)  [unwired: 1 in]
                    n2682 = Decrement(x=w3216) -> (x-1=w3215:i32)
                    n2683 = Replace Array Subset(array=bool[] [FALSE, FALSE, FALSE, FALSE, FALSE, FALSE, FALSE, FALSE, FALSE, FALSE, FALSE, FALSE, FALSE, FALSE, FALSE, FALSE, FALSE, FALSE, FALSE, FALSE, FALSE, FALSE, FALSE, FALSE, FALSE, FALSE, FALSE, FALSE, FALSE, FALSE, FALSE, FALSE, FALSE, FALSE, FALSE, FALSE, FALSE, FALSE, FALSE, FALSE, FALSE, FALSE, FALSE, FALSE, FALSE, FALSE, FALSE, FALSE, FALSE, FALSE, FALSE, FALSE, FALSE, FALSE, FALSE, FALSE, FALSE, FALSE, FALSE, FALSE, FALSE, FALSE, FALSE, FALSE, FALSE, FALSE, FALSE, FALSE, FALSE, FALSE, FALSE, FALSE, FALSE, FALSE, FALSE, FALSE, FALSE, FALSE, FALSE, FALSE, FALSE, FALSE, FALSE, FALSE, FALSE, FALSE, FALSE, FALSE, FALSE, FALSE, FALSE, FALSE, FALSE, FALSE, FALSE, FALSE, FALSE, FALSE, FALSE, FALSE, FALSE, FALSE, FALSE, FALSE, FALSE, FALSE, FALSE, FALSE, FALSE, FALSE, FALSE, FALSE, FALSE, FALSE, FALSE, FALSE, FALSE, FALSE, FALSE, FALSE, FALSE, FALSE, FALSE, FALSE, FALSE, FALSE, FALSE, FALSE, FALSE, FALSE, FALSE, FALSE, FALSE, FALSE, FALSE, FALSE, FALSE, FALSE, FALSE, FALSE, FALSE, FALSE, FALSE, FALSE, FALSE, FALSE, FALSE, FALSE, FALSE, FALSE, FALSE, FALSE, FALSE, FALSE, FALSE, FALSE, FALSE, FALSE, FALSE, FALSE, FALSE, FALSE, FALSE, FALSE, FALSE, FALSE, FALSE, FALSE, FALSE, FALSE, FALSE, FALSE, FALSE, FALSE, FALSE, FALSE, FALSE, FALSE, FALSE, FALSE, FALSE, FALSE, FALSE, FALSE, FALSE, FALSE, FALSE, FALSE, FALSE, FALSE, FALSE, FALSE, FALSE, FALSE, FALSE, FALSE, FALSE, FALSE, FALSE, FALSE] ("appended array"), new element=TRUE, index=w3215) -> (w3213:bool[])
                    n2684 = Array Subset(array=w3213, length=w3212) -> (w3211:bool[])  [unwired: 1 in]
                    n2685 = Array Subset(array=w3213, index=w3212, length=w3212) -> (w3210:bool[])
                    n2686 = Array To Cluster(array=w3211) -> (cluster=w3209:T48)
                    n2687 = Array To Cluster(array=w3210) -> (cluster=w3208:T48)
                    n2688 = Build Array(w3209, w3208) -> (w3207:T55)
                    n2689 = property on="UEAArray" class="Arr (strict)"("Val(Sgnl)"=w3207) -> ()  [unwired: 2 in, 2 out]
                  }
                  frame "Right" {
                    w3231 = 100 ("length")
                    n2690 = local read "EncodeClust"() -> (w3244:T9)
                    n2691 = Unbundle By Name(w3244) -> ("UEAArray"=w3239:T25)
                    n2692 = Index Array(array=w3239) -> (element #1=w3240:T54, element #2=w3241:T54)  [unwired: 2 in]
                    n2693 = Cluster To Array(cluster=w3240) -> (array=w3242:bool[])
                    n2694 = Cluster To Array(cluster=w3241) -> (array=w3243:bool[])
                    n2695 = Build Array (concatenate)(w3242, w3243) -> (w3238:bool[])
                    n2696 = Search 1D Array(1D array=w3238, element=TRUE) -> (index of element=w3235:i32)  [unwired: 1 in]
                    n2697 = Increment(x=w3235) -> (x+1=w3234:i32)
                    n2698 = Replace Array Subset(array=bool[] [FALSE, FALSE, FALSE, FALSE, FALSE, FALSE, FALSE, FALSE, FALSE, FALSE, FALSE, FALSE, FALSE, FALSE, FALSE, FALSE, FALSE, FALSE, FALSE, FALSE, FALSE, FALSE, FALSE, FALSE, FALSE, FALSE, FALSE, FALSE, FALSE, FALSE, FALSE, FALSE, FALSE, FALSE, FALSE, FALSE, FALSE, FALSE, FALSE, FALSE, FALSE, FALSE, FALSE, FALSE, FALSE, FALSE, FALSE, FALSE, FALSE, FALSE, FALSE, FALSE, FALSE, FALSE, FALSE, FALSE, FALSE, FALSE, FALSE, FALSE, FALSE, FALSE, FALSE, FALSE, FALSE, FALSE, FALSE, FALSE, FALSE, FALSE, FALSE, FALSE, FALSE, FALSE, FALSE, FALSE, FALSE, FALSE, FALSE, FALSE, FALSE, FALSE, FALSE, FALSE, FALSE, FALSE, FALSE, FALSE, FALSE, FALSE, FALSE, FALSE, FALSE, FALSE, FALSE, FALSE, FALSE, FALSE, FALSE, FALSE, FALSE, FALSE, FALSE, FALSE, FALSE, FALSE, FALSE, FALSE, FALSE, FALSE, FALSE, FALSE, FALSE, FALSE, FALSE, FALSE, FALSE, FALSE, FALSE, FALSE, FALSE, FALSE, FALSE, FALSE, FALSE, FALSE, FALSE, FALSE, FALSE, FALSE, FALSE, FALSE, FALSE, FALSE, FALSE, FALSE, FALSE, FALSE, FALSE, FALSE, FALSE, FALSE, FALSE, FALSE, FALSE, FALSE, FALSE, FALSE, FALSE, FALSE, FALSE, FALSE, FALSE, FALSE, FALSE, FALSE, FALSE, FALSE, FALSE, FALSE, FALSE, FALSE, FALSE, FALSE, FALSE, FALSE, FALSE, FALSE, FALSE, FALSE, FALSE, FALSE, FALSE, FALSE, FALSE, FALSE, FALSE, FALSE, FALSE, FALSE, FALSE, FALSE, FALSE, FALSE, FALSE, FALSE, FALSE, FALSE, FALSE, FALSE, FALSE, FALSE, FALSE, FALSE, FALSE, FALSE, FALSE, FALSE, FALSE, FALSE] ("appended array"), new element=TRUE, index=w3234) -> (w3232:bool[])
                    n2699 = Array Subset(array=w3232, length=w3231) -> (w3230:bool[])  [unwired: 1 in]
                    n2700 = Array Subset(array=w3232, index=w3231, length=w3231) -> (w3229:bool[])
                    n2701 = Array To Cluster(array=w3230) -> (cluster=w3228:T48)
                    n2702 = Array To Cluster(array=w3229) -> (cluster=w3227:T48)
                    n2703 = Build Array(w3228, w3227) -> (w3226:T55)
                    n2704 = property on="UEAArray" class="Arr (strict)"("Val(Sgnl)"=w3226) -> ()  [unwired: 2 in, 2 out]
                  }
                }
              }
            }
          }
          event "ManualClust": Mouse Down {
            n2705 = event-data() -> ("Mods"=w3247:cluster{"Double Click":bool, "Menu Key":bool})  [unwired: 1 in, 7 out]
            n2706 = Unbundle By Name(w3247) -> ("Double Click"=w3245:bool)
            n2707 = case shown="True" w3245 {
              frame False {
              }
              frame True {
                n2708 = local write "ManualClust"(T7 {"Thumb"=0.0, "Index"=0.0, "Middle"=0.0, "Ring"=0.0, "Little"=0.0, "ThumbInt"=0.0, "IndexInt"=0.0, "RingInt"=0.0, "LittleInt"=0.0, "WristPitch"=0.0, "WristYaw"=0.0, "WristRoll"=0.0} ("ManualClust")) -> ()
              }
            }
          }
        }
      }
      n2709 = node-c288(w329) -> ()  [unwired: 1 out]
    }
    frame #2 {
      n2710 = stacked-sequence {
        frame #0 {
          # "Writing initial trial parameters to txt file and NIP"
          # "need to add an entry to TrialArray in case program finishes without running a trial (see RippleEMG)"
          n2711 = local read "MvntBuilder"() -> (w3886:T6)
          n2712 = local read "Timing"() -> (w3888:T3)
          n2713 = local read "CurrMvnt"() -> (w3885:T1)
          n2714 = Unbundle By Name(w3886) -> ("TargParams"=w3887:cluster{"Gain":dbl, "Radius":dbl, "Acc":dbl})
          n2715 = local read "DecodeClust"() -> (w3891:T5)
          n2716 = local read "TrialArray"() -> (w3889:string[])
          n2717 = local read "NIPTime"() -> (w3883:dbl)
          n2718 = call "FeedbackDecode_FPPNS2NIP.vi"("NIPTime"=w3883, "LoopCnt"=-1, "DecodeClust"=w3891, "TrialTiming"=w3888, "TargParams"=w3887, "MvntClust"=w3885) -> ("TrialParams"=w3890:string)  [unwired: 5 in]
          n2719 = local read "EventParamsFID"() -> (w3884:refnum<file>)
          n2720 = Insert Into Array(array=w3889, new element=w3890) -> (w3892:string[])  [unwired: 1 in]
          n2721 = local write "TrialArray"(w3892) -> ()
          n2722 = call "FeedbackDecode_WriteTextEOL.vi"("text"=w3890, "refnum in"=w3884) -> ()  [unwired: 8 in, 2 out]
        }
        frame #1 {
          w3896 = "_" ("string")
          w3898 = ".txt" ("string")
          # "Save Params and Preset Tables"
          n2723 = local read "DecodeClust"() -> (w3895:T5)
          n2724 = Unbundle By Name(w3895) -> ("DataFolder"=w3894:string)
          n2725 = Get Date/Time In Seconds() -> (seconds since 1Jan1904=w3907:timestamp)
          n2726 = Format Date/Time String(time format string (%c)="%H%M%S", seconds (now)=w3907) -> (date/time string=w3899:string)  [unwired: 1 in]
          n2727 = local read "EncodeClust"() -> (w3900:T9)
          n2728 = local read "DataPath"() -> (w3897:path)
          n2729 = Concatenate Strings("StimParams_" ("name or relative path"), w3894, w3896, w3899, w3898) -> (w3905:string)
          n2730 = Unbundle By Name(w3900) -> ("ParamsTable"=w3909:string[][])
          n2731 = Build Path(base path=w3897, name or relative path=w3905) -> (appended path=w3904:path)
          n2732 = Unbundle By Name(w3900) -> ("PresetTable"=w3893:string[][])
          n2733 = call-poly <vilib>:"Write Delimited Spreadsheet.vi"("file path (dialog if empty)"=w3904, "2D data"=w3909) -> ()  [unwired: 12 in, 2 out]
          n2734 = Concatenate Strings("StimPresets_" ("name or relative path"), w3894, w3896, w3899, w3898) -> (w3902:string)
          n2735 = Build Path(base path=w3897, name or relative path=w3902) -> (appended path=w3901:path)
          n2736 = call-poly <vilib>:"Write Delimited Spreadsheet.vi"("file path (dialog if empty)"=w3901, "2D data"=w3893) -> ()  [unwired: 12 in, 2 out]
        }
        frame #2 {
          # "Stopping NIP recording and moving unnamed data files into the appropriate data folder on drive D:"
          n2737 = local read "DecodeClust"() -> (w3916:T5)
          n2738 = Bundle By Name(cluster=w3916, "EventStr"="SS.Stop=1;") -> (w3913:T5)
          n2739 = call "FeedbackDecode_MLComCtrl.vi"("DecodeClustIn"=w3913, "Mode"=T19."SendEvent") -> ("DecodeClustOut"=w3912:T5)  [unwired: 6 in, 3 out]
          n2740 = call "FeedbackDecode_MLComCtrl.vi"("DecodeClustIn"=w3912, "Mode"=T19."Wait") -> ("DecodeClustOut"=w3911:T5)  [unwired: 6 in, 3 out]
          n2741 = Bundle By Name(cluster=w3911, "CtrlButtons.Stop"=FALSE) -> (w3910:T5)
          n2742 = local write "DecodeClust"(w3910) -> ()
        }
        frame #3 {
          # "Copy files from RemoteRepo on Matlab computer"
          n2743 = local read "DecodeClust"() -> (w3919:T5)
          n2744 = Unbundle By Name(w3919) -> ("NumComp"=w3920:enum16{"1 Computer", "2 Computers"})
          n2745 = case shown="\"2 Computers\", Default" w3920 {
            tunnel: w3919 -> [_ w3921]
            frame "1 Computer" {
            }
            frame "2 Computers", Default {
              n2746 = call "FeedbackDecode_MLComCtrl.vi"("DecodeClustIn"=w3921, "Mode"=T19."CopyTraining") -> ()  [unwired: 6 in, 4 out]
            }
          }
        }
        frame #4 {
          n2747 = call "Data options"() -> ("Delete from D drive?"=→"Delete from D drive?":bool, "Copy to raid?"=→"Copy to raid?":bool, "Don't save to database?"=→"Don't save to database?":bool)  [unwired: 15 in, 2 out]
        }
        frame #5 {
          # "add to database"
          n2748 = local read "Don't save to database?"() -> (w3926:bool)
          n2749 = case shown="False" w3926 {
            frame False {
              n2750 = local read "DecodeClust"() -> (w3928:T5)
              n2751 = local read "ExperimentDate"() -> (w3934:timestamp)
              n2752 = local read "TaskType"() -> (w3933:string)
              n2753 = Unbundle By Name(w3928) -> ("DataFolder"=w3927:string)
              n2754 = Empty String/Path?(string/path=w3927) -> (empty?=w3929:bool)
              n2755 = local read "Database"() -> (w3935:T12)
              n2756 = Bundle By Name(cluster=w3935, "ExperimentDate"=w3934, "CerebusFolder"=w3927, "TaskType"=w3933) -> (w3930:T12)
              n2757 = case shown="True" w3929 {
                frame False {
                }
                frame True {
                  n2758 = One Button Dialog(message="The data folder is unknown and will not be saved to the database. Make sure to update the database manually with the appropriate folder name!") -> ()  [unwired: 1 in, 1 out]
                }
              }
              n2759 = local read "DatabaseUDL"() -> (w3932:path)
              n2760 = local write "Database"(w3930) -> ()
              n2761 = call "FeedbackDecode_UpdateDatabase.vi"("DatabaseIn"=w3930, "CallType"=enum16{"Initialize", "Save", "Load"}."Save", "DatabaseUDL"=w3932) -> ()  [unwired: 1 in, 3 out]
            }
            frame True {
            }
          }
        }
        frame #6 {
          # "copy to raid"
          n2762 = flat-sequence {
            frame #0 {
              "CopySucc" <- FALSE
            }
            frame #1 {
              n2763 = local read "Copy to raid?"() -> (w3938:bool)
              n2764 = case shown="True" w3938 {
                frame False {
                }
                frame True {
                  n2765 = local read "DecodeClust"() -> (w3943:T5)
                  n2766 = local read "Database"() -> (w3942:T12)
                  n2767 = Unbundle By Name(w3942) -> ("PatientNumber"=w3939:string)
                  n2768 = Unbundle By Name(w3943) -> ("DataFolder"=w3941:string)
                  n2769 = Empty String/Path?(string/path=w3939) -> (empty?=w3940:bool)
                  n2770 = case shown="False" w3940 {
                    tunnel: w3941 -> [w3951 _]
                    tunnel: w3939 -> [w3949 _]
                    frame False {
                      n2771 = Concatenate Strings("E:\\Data\\" ("string"), w3949, "\\" ("string"), w3951) -> (w3952:string)
                      n2772 = String To Path(string=w3952) -> (path=w3944:path)
                      n2773 = Strip Path(path=w3944) -> (stripped path=w3945:path)  [unwired: 1 out]
                      n2774 = call <vilib>:"Check if File or Folder Exists.vi"("path"=w3945) -> ("error out"=w3947:errorcluster, "file or folder exists?"=w3946:bool)  [unwired: 8 in, 1 out]
                      n2775 = case shown="True" w3946 {
                        tunnel: w3947 -> [_ w3956]
                        tunnel: w3944 -> [_ w3957]
                        frame False {
                          n2776 = One Button Dialog(message="Cannot copy to raid. Patient folder does not exist on raid.") -> ()  [unwired: 1 in, 1 out]
                        }
                        frame True {
                          n2777 = local read "DataPath"() -> (w3958:path)
                          n2778 = Copy(8:w3956, 10:w3957, 11:w3958) -> (1:w3955:bool)  [unwired: 2 in, 2 out]
                          n2779 = Not(x=w3955) -> (.not. x?=w3954:bool)
                          n2780 = local write "CopySucc"(w3954) -> ()
                        }
                      }
                    }
                    frame True {
                      n2781 = One Button Dialog(message="Cannot copy to raid. Patient number is missing in database.") -> ()  [unwired: 1 in, 1 out]
                    }
                  }
                }
              }
            }
          }
        }
        frame #7 {
          w3963 = FALSE ("Blinking")
          n2782 = local read "RespRefArray"() -> (w3962:refnum<vi>[])
          n2783 = disable-structure shown="Disabled" {
            frame Disabled {
              n2784 = vi-ref "FeedbackDecode_MSMS2DEKA.vi"() -> (w3977:refnum<vi>)
              n2785 = property class="VI"(reference=w3977) -> (reference out=w3975:refnum<vi>, "FP.State"=w3976:T21)  [unwired: 1 in, 1 out]
              n2786 = case shown="\"Standard\", Default" w3976 {
                tunnel: w3975 -> [_ w3978]
                frame "Closed" {
                }
                frame "Standard", Default {
                  n2787 = invoke class="VI" method="FP.Close"(reference=w3978) -> ()  [unwired: 2 in, 3 out]
                }
              }
            }
            frame Enabled {
            }
          }
          n2788 = for {
            tunnel: w3962 -> [w3979] mode=indexing
            n2789 = property class="VI"(reference=w3979) -> (reference out=w3981:refnum<vi>, "FP.State"=w3980:T21)  [unwired: 1 in, 1 out]
            n2790 = case shown="\"Standard\", Default" w3980 {
              tunnel: w3981 -> [_ w3982]
              frame "Closed" {
              }
              frame "Standard", Default {
                n2791 = invoke class="VI" method="FP.Close"(reference=w3982) -> ()  [unwired: 2 in, 3 out]
              }
            }
          }
          n2792 = disable-structure shown="Disabled" {
            frame Disabled {
              n2793 = vi-ref "FeedbackDecode_AllEMGHM.vi"() -> (w3983:refnum<vi>)
              n2794 = invoke class="VI" method="FP.Close"(reference=w3983) -> ()  [unwired: 2 in, 3 out]
            }
            frame Enabled {
            }
          }
          n2795 = local write "LVTab"(enum32{"Decode", "Encode", "Video", "Database"}."Decode" ("LVTab")) -> ()
          n2796 = local read "EncodeClust"() -> (w3965:T9)
          n2797 = local read "DecodeClust"() -> (w3968:T5)
          n2798 = local read "EventParamsFID"() -> (w3969:refnum<file>)
          n2799 = local read "PSRef"() -> (w3973:refnum<vi>)
          n2800 = Close Reference(reference=w3973) -> ()  [unwired: 1 in, 1 out]
          n2801 = call "FeedbackDecode_MLComCtrl.vi"("DecodeClustIn"=w3968, "EncodeClustIn"=w3965, "Mode"=T19."Close") -> ("DecodeClustOut"=w3967:T5, "EncodeClustOut"=w3966:T9)  [unwired: 5 in, 2 out]
          n2802 = call "FeedbackDecode_SendMSMSPacket.vi"("Mode"=enum16{"Initialize", "Run", "Close"}."Close") -> ()  [unwired: 6 in]
          n2803 = Close File(refnum=w3969) -> ()  [unwired: 1 in, 2 out]
          n2804 = local write "EncodeClust"(w3966) -> ()
          n2805 = local write "DecodeClust"(w3967) -> ()
          n2806 = local read "DAQmx?"() -> (w3960:bool)
          n2807 = case shown="True" w3960 {
            frame False {
            }
            frame True {
              n2808 = call <vilib>:"DAQmx Stop Task.vi"("task/channels in"=refnum<k21> "AO0") -> ()  [unwired: 13 in, 2 out]
            }
          }
          n2809 = global write "FeedbackDecode_Globals.vi" "FD_Stop"(FALSE ("G_Stop")) -> ()
          n2810 = property on="Finished" class="Bool (strict)"("DisabledEnum"=T17."Disabled and Grayed Out" ("Disabled"), "Blinking"=w3963, "Value"=w3963) -> ()  [unwired: 2 in, 2 out]
        }
        frame #8 {
          n2811 = local read "Delete from D drive?"() -> (w3984:bool)
          n2812 = case shown="True" w3984 {
            frame False {
            }
            frame True {
              n2813 = local read "CopySucc"() -> (w3985:bool)
              n2814 = case shown="False" w3985 {
                frame False {
                  n2815 = Two Button Dialog(message="Data was not copied to raid. Delete anyway? ", 2:"Yes" ("T button name (\"OK\")")) -> (T button?=w3986:bool)  [unwired: 1 in]
                  n2816 = case shown="True" w3986 {
                    frame False {
                    }
                    frame True {
                      w3989 = TRUE ("confirm (F)")
                      n2817 = local read "DataPath"() -> (w3990:path)
                      n2818 = Delete(path (use dialog)=w3990, entire hierarchy (F)=w3989, confirm (F)=w3989) -> ()  [unwired: 2 in, 3 out]
                    }
                  }
                }
                frame True {
                  w3991 = TRUE ("confirm (F)")
                  n2819 = local read "DataPath"() -> (w3992:path)
                  n2820 = Delete(path (use dialog)=w3992, entire hierarchy (F)=w3991, confirm (F)=w3991) -> ()  [unwired: 2 in, 3 out]
                }
              }
            }
          }
        }
      }
    }
  }
